vi "ManualControls_v4.vi"() -> ()   [LabVIEW 2013]
uses:
  <vilib>/Utility/miscctls.llb/LVPointTypeDef.ctl
  <vilib>/DAQmx/write.llb/DAQmx Write (Analog DBL 1Chan 1Samp).vi
  <vilib>/DAQmx/write.llb/DAQmx Write (Digital U32 1Chan 1Samp).vi
  <vilib>/DAQmx/miscellaneous.llb/DAQmx Fill In Error Info.vi
  DeviceVIs/Novatech/Novatech 409A.lvlib
panel:
  in  "Update Hardware":bool
  in  "?":enum32{"Controls", "File IO", "Errors"}(tab)
  in  "Master Output Bits":bool[](array[boolean])=[TRUE, TRUE, TRUE, TRUE, FALSE, FALSE, TRUE, FALSE, FALSE, FALSE, TRUE, FALSE, TRUE, TRUE, TRUE, TRUE, FALSE, FALSE, FALSE, FALSE, FALSE, FALSE, FALSE, FALSE]
  in  "Slave Output Bits":bool[](array[boolean])=[FALSE, FALSE, FALSE, FALSE, FALSE, FALSE, FALSE, FALSE, FALSE, FALSE, FALSE, FALSE, FALSE, FALSE, FALSE, FALSE, FALSE, FALSE, FALSE, FALSE, FALSE, FALSE, FALSE, FALSE]
  in  "Set Master":bool=TRUE
  in  "Set Slave":bool
  in  "AO Values":T1(array[cluster])=[{"DAQmx Global Channel"="AO0_0", "Numeric"=-9.792}, {"DAQmx Global Channel"="AO0_1", "Numeric"=-7.904}, {"DAQmx Global Channel"="AO0_2", "Numeric"=-3.981}, {"DAQmx Global Channel"="AO0_3", "Numeric"=-7.5}, {"DAQmx Global Channel"="AO0_4", "Numeric"=7.0}, {"DAQmx Global Channel"="AO0_5", "Numeric"=1.18}, {"DAQmx Global Channel"="AO0_6", "Numeric"=-8.918}, {"DAQmx Global Channel"="AO0_7", "Numeric"=1.1}, {"DAQmx Global Channel"="AO1_0", "Numeric"=8.0}, {"DAQmx Global Channel"="AO1_1", "Numeric"=0.45}, {"DAQmx Global Channel"="AO1_2", "Numeric"=1.3}, {"DAQmx Global Channel"="AO1_3", "Numeric"=0.0}, {"DAQmx Global Channel"="AO1_4", "Numeric"=0.3}, {"DAQmx Global Channel"="AO1_5", "Numeric"=1.2}, {"DAQmx Global Channel"="AO1_6", "Numeric"=1.6}, {"DAQmx Global Channel"="AO1_7", "Numeric"=0.12}, {"DAQmx Global Channel"="AO2_0", "Numeric"=0.0}, {"DAQmx Global Channel"="AO2_1", "Numeric"=0.0}, {"DAQmx Global Channel"="AO3_0", "Numeric"=0.0}, {"DAQmx Global Channel"="AO3_1", "Numeric"=0.0}, {"DAQmx Global Channel"="AO3_2", "Numeric"=0.0}, {"DAQmx Global Channel"="AO3_3", "Numeric"=0.0}, {"DAQmx Global Channel"="AO3_4", "Numeric"=0.0}, {"DAQmx Global Channel"="AO3_5", "Numeric"=0.0}, {"DAQmx Global Channel"="AO3_6", "Numeric"=0.0}, {"DAQmx Global Channel"="AO3_7", "Numeric"=0.0}] {"Numeric" step=1e-09 format="%_6g"}
  in  "Presets":T2(ring)
  in  "DO Values":T3(array[cluster])=[{"DAQmx Global Channel"="DO0_0", "DO Bits"=[TRUE, TRUE, FALSE, FALSE, FALSE, FALSE, TRUE, TRUE, FALSE, FALSE, FALSE, FALSE, FALSE, FALSE, FALSE, FALSE]}, {"DAQmx Global Channel"="DO1_0", "DO Bits"=[TRUE, FALSE, TRUE, TRUE, FALSE, TRUE, TRUE, TRUE, FALSE, FALSE, FALSE, FALSE, FALSE, FALSE, FALSE, FALSE]}, {"DAQmx Global Channel"="DO2_0", "DO Bits"=[]}, {"DAQmx Global Channel"="DO3_0", "DO Bits"=[]}]
  in  "Novatech settings":T4(array[cluster])
  in  "History":string(combo)
  in  "Save":bool
  in  "Load":bool
  in  "Path":path=path "C:/Experiment/Data Acquisition/Hardware Control/procedures/ManualControl"
  in  "error in":errorcluster
  out "error out":errorcluster
  # "Analog out"
  # "Digital Out"
  # "Ports are setup for 16 bit output, but only 16 are used"
  # "Master PB (PB 0)"
  # "Slave PB (PB 1)"
  # "Novatechs"
  # "0"
  # "8"
  # "12"
  # "4"
  # "16"
  # "20"
  # "0"
  # "8"
  # "12"
  # "4"
  # "16"
  # "20"
  # "Templates"
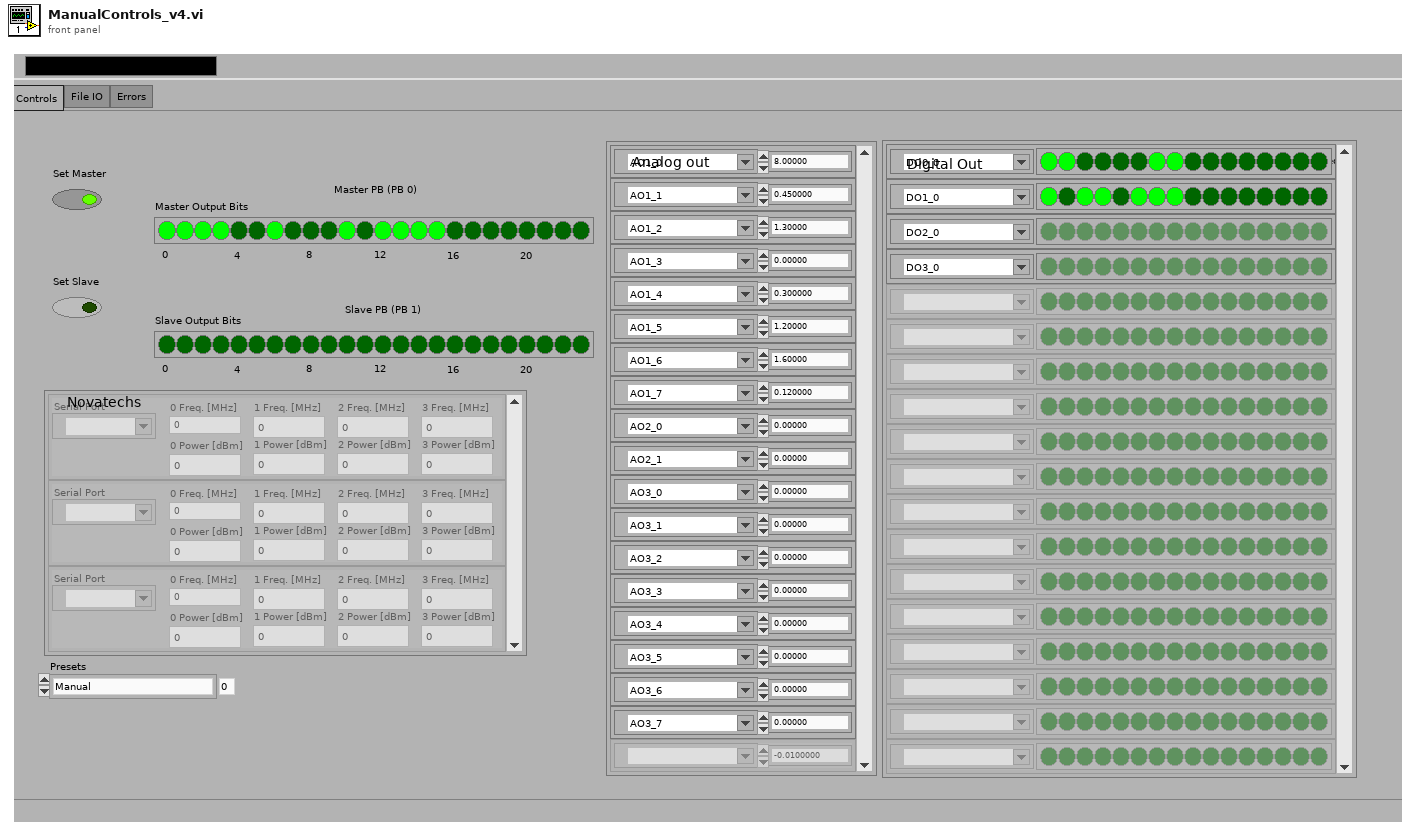
[diagram p1: front panel]
types:
  T1 = cluster{"DAQmx Global Channel":refnum<k21>, "Numeric":dbl}[]
  T2 = enum16{"Manual", "Rb MOT", "Yb MOT", "RbYb Warmup", "RbYb Turn Off", "Sr Warmup"}
  T3 = cluster{"DAQmx Global Channel":refnum<k21>, "DO Bits":bool[]}[]
  T4 = cluster{"0 Freq. [MHz]":dbl, "0 Power [dBm]":dbl, "Serial Port":refnum<visa-resource-name>, "1 Freq. [MHz]":dbl, "1 Power [dBm]":dbl, "2 Freq. [MHz]":dbl, "2 Power [dBm]":dbl, "3 Freq. [MHz]":dbl, "3 Power [dBm]":dbl}[]
  T5 = typedef "Semaphore RefNum" = refnum<k1>
  T6 = enum16{"open", "open or create", "create or replace", "create", "open (read only)"}
  T7 = enum16{"Always On", "Always Off", "Off While Running"}
  T8 = typedef "LVPointTypeDef.ctl" = cluster{"Horizontal":i16, "Vertical":i16}
  T9 = cluster{"Master Output Bits":bool[], "Slave Output Bits":bool[], "AO Values":cluster{"DAQmx Global Channel":refnum<k21>, "Numeric":dbl}[], "DO Values":cluster{"DAQmx Global Channel":refnum<k21>, "DO Bits":bool[]}[], "Novatech settings":cluster{"0 Freq. [MHz]":dbl, "0 Power [dBm]":dbl, "Serial Port":refnum<visa-resource-name>, "1 Freq. [MHz]":dbl, "1 Power [dBm]":dbl, "2 Freq. [MHz]":dbl, "2 Power [dBm]":dbl, "3 Freq. [MHz]":dbl, "3 Power [dBm]":dbl}[]}
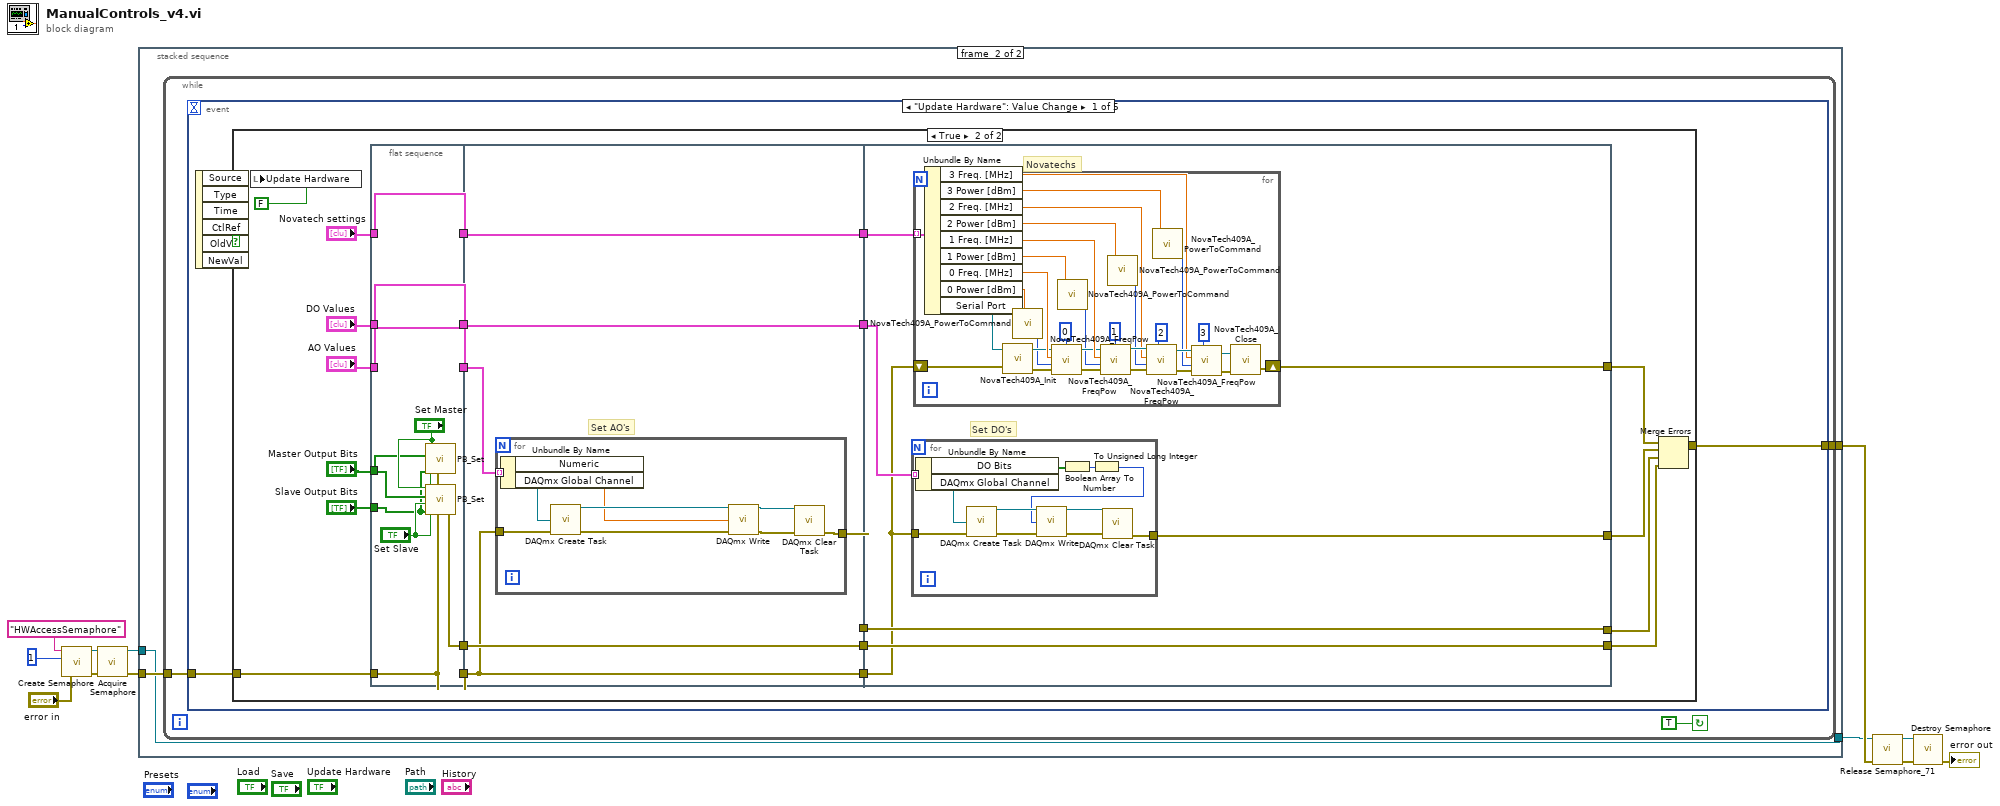
[diagram p0: block diagram]
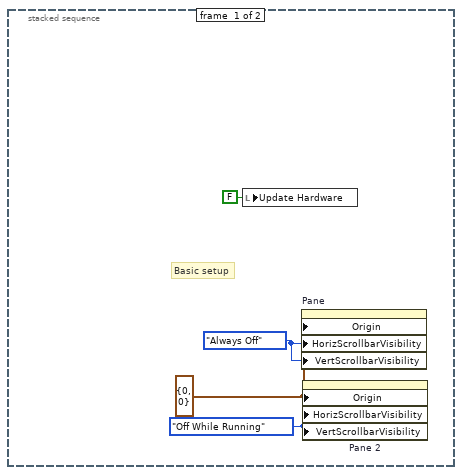
[diagram p2: hidden frame]
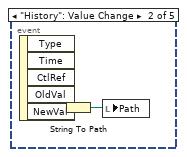
[diagram p4: hidden frame]
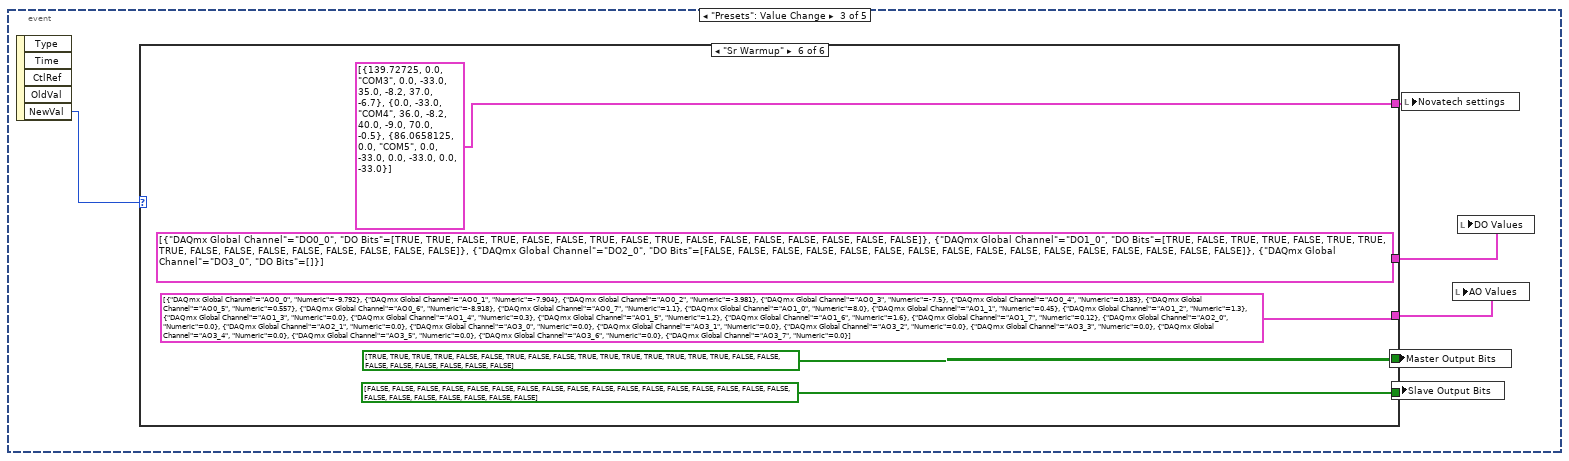
[diagram p5: hidden frame]
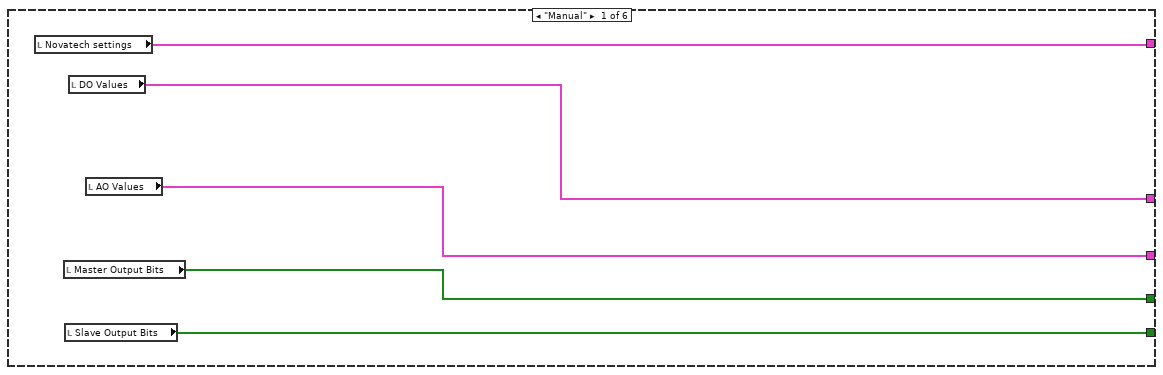
[diagram p6: hidden frame]
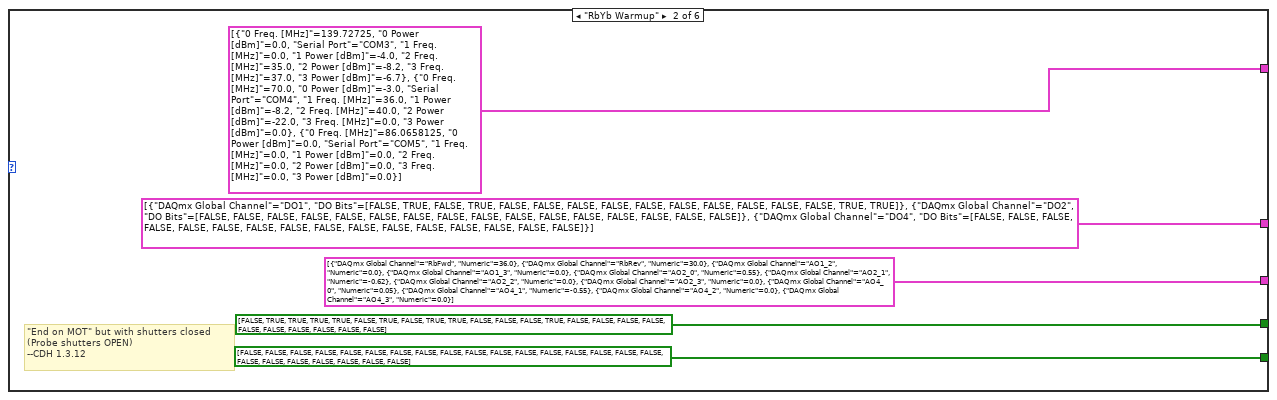
[diagram p7: hidden frame]
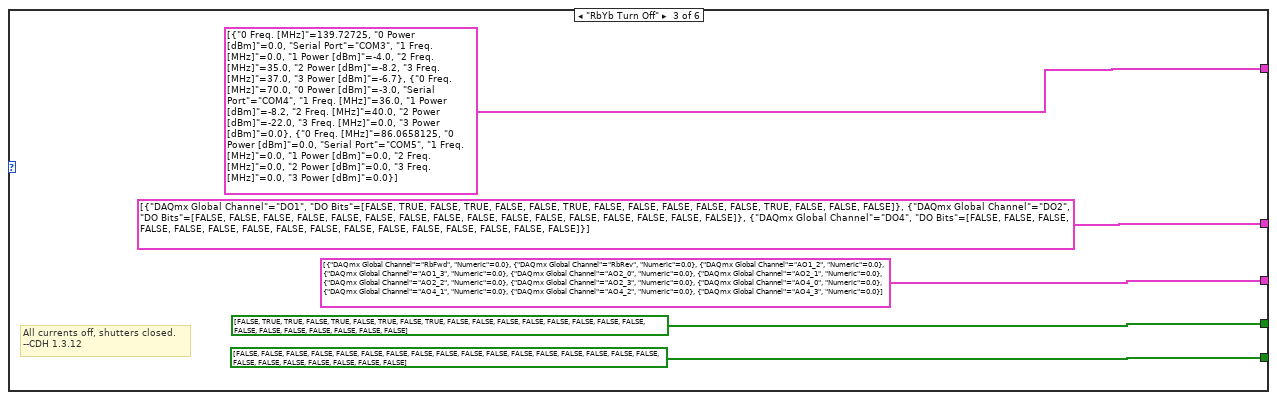
[diagram p8: hidden frame]
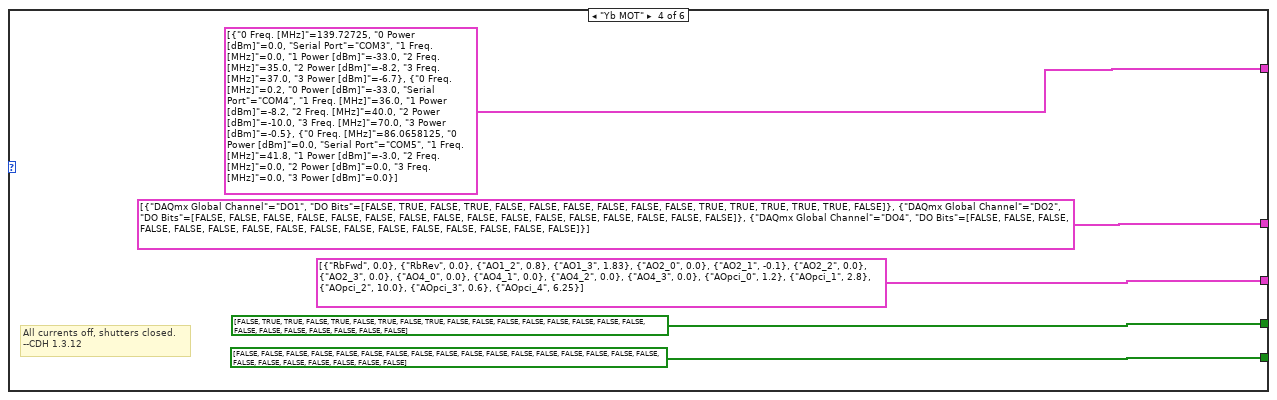
[diagram p9: hidden frame]
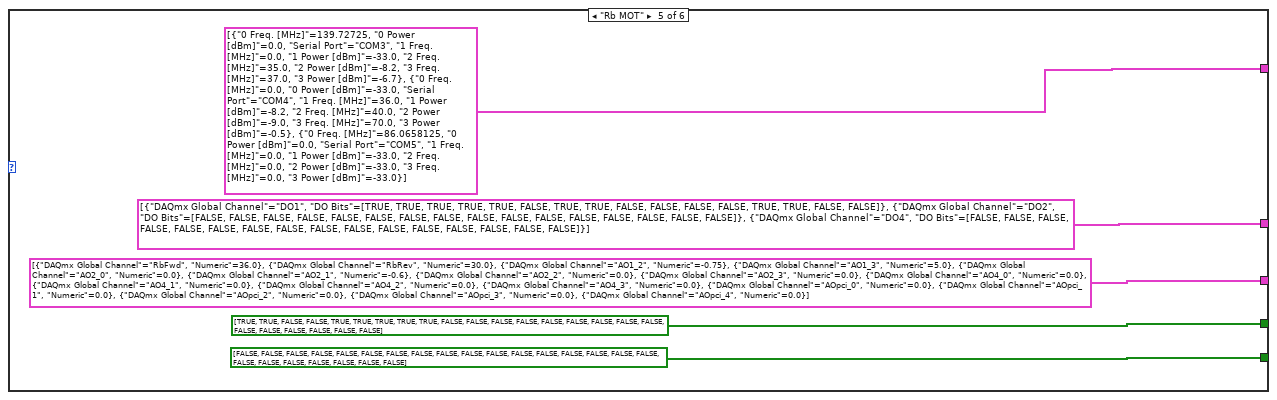
[diagram p10: hidden frame]
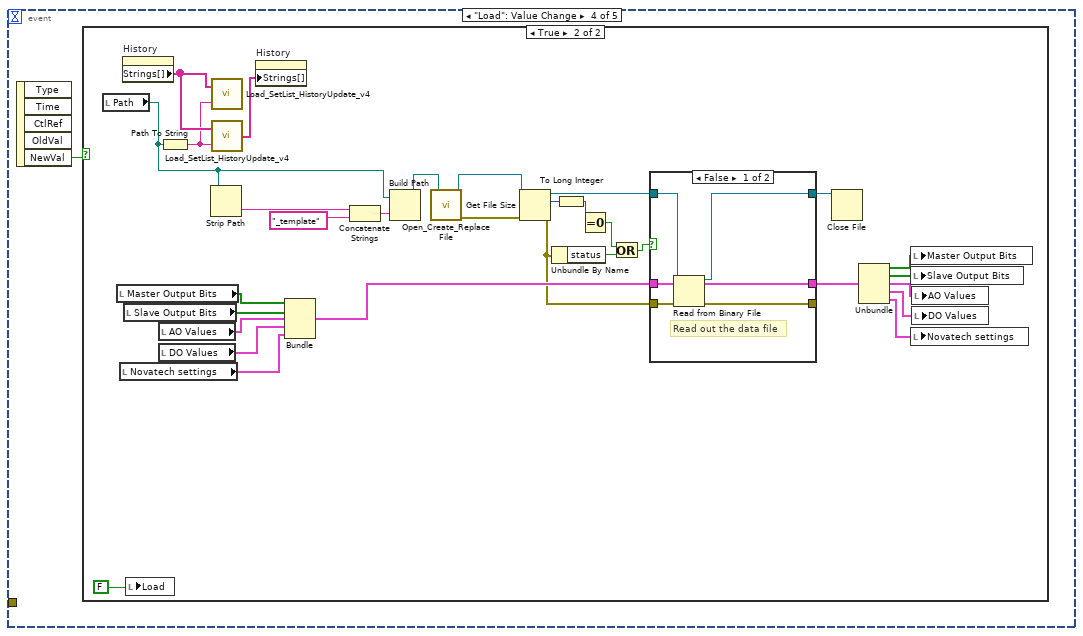
[diagram p11: hidden frame]
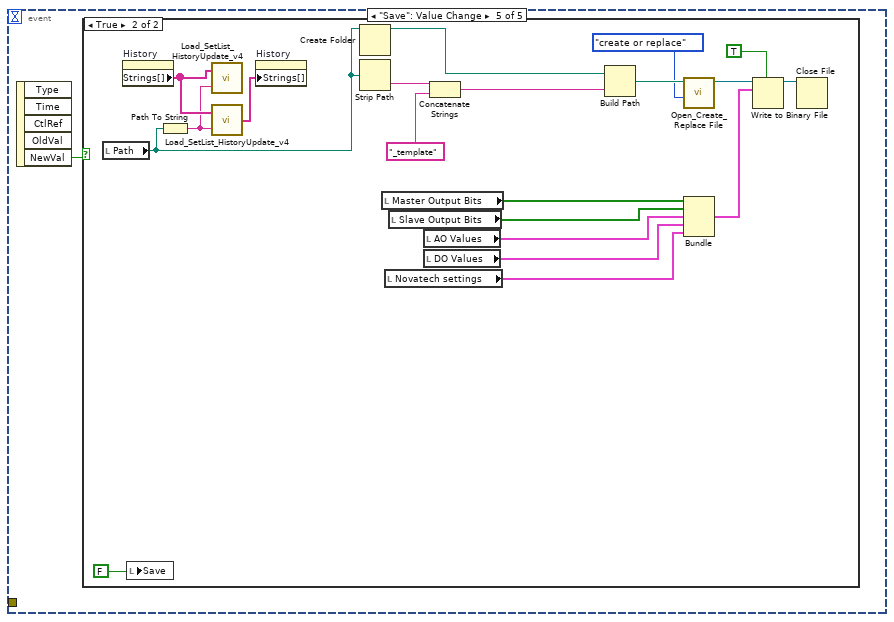
[diagram p14: hidden frame]
diagram:
  n1 = call <vilib>:"Create Semaphore.vi"("error in (no error)"="error in", "size (1)"=1, "name (unnamed)"="HWAccessSemaphore") -> ("error out"=w6:errorcluster, "semaphore"=w7:T5)  [unwired: 3 out]
  n2 = call <vilib>:"Acquire Semaphore.vi"("error in (no error)"=w6, "semaphore"=w7) -> ("error out"=w3:errorcluster, "semaphore out"=w2:T5)  [unwired: 1 in, 3 out]
  n3 = stacked-sequence {
    tunnel: [_ w19] -> w9
    tunnel: w3 -> [_ w18]
    tunnel: w2 -> [_ w17]
    tunnel: [_ w17] -> w1
    frame #0 {
      w16 = T7."Always Off" ("Horizontal Scrollbar Visibility")
      w15 = T8 {"Horizontal"=0, "Vertical"=0} ("Origin")
      w14 = T7."Off While Running" ("Horizontal Scrollbar Visibility")
      # "Basic setup"
      n4 = local write "Update Hardware"(FALSE ("Update Hardware")) -> ()
      n5 = property on="Pane" class="Pane"("Origin"=w15, "HorizScrollbarVisibility"=w16, "VertScrollbarVisibility"=w16) -> ()  [unwired: 2 in, 2 out]
      n6 = property on="Pane 2" class="Pane"("Origin"=w15, "HorizScrollbarVisibility"=w14, "VertScrollbarVisibility"=w14) -> ()  [unwired: 2 in, 2 out]
    }
    frame #1 {
      n7 = while {
        tunnel: [w22] -> w19
        tunnel: w18 -> [w21]
        stop <- TRUE continue-if-true
        n8 = event shown="[0] \"Update Hardware\": Value Change" {
          selector: _ -> [_ _ _ _ _]
          dyn-events: _ -> [_ _ _ _ _]
          timeout: _ -> [_ _ _ _ _]
          tunnel: [w25 _ _ _ _] -> w22
          tunnel: w21 -> [w24 _ _ _ _]
          event "Update Hardware": Value Change {
            n9 = event-data() -> ("OldVal"=w23:bool)  [unwired: 1 in, 5 out]
            n10 = case shown="True" w23 {
              tunnel: [w26 w36] -> w25
              tunnel: w24 -> [w26 w35]
              frame False {
              }
              frame True {
                n11 = local write "Update Hardware"(FALSE) -> ()
                n12 = flat-sequence {
                  tunnel: [w49] -> w48
                  tunnel: [w55] -> w47
                  tunnel: "AO Values" -> [w55]
                  tunnel: "Master Output Bits" -> [w54]
                  tunnel: "Slave Output Bits" -> [w53]
                  tunnel: "DO Values" -> [w51]
                  tunnel: "Novatech settings" -> [w52]
                  tunnel: [w51] -> w46
                  tunnel: [w52] -> w45
                  tunnel: w35 -> [w50]
                  tunnel: [w50] -> w44
                  tunnel: w48 -> [w59]
                  tunnel: w47 -> [w62]
                  tunnel: [w63] -> w43
                  tunnel: w46 -> [w61]
                  tunnel: [w61] -> w42
                  tunnel: [w60] -> w41
                  tunnel: w45 -> [w60]
                  tunnel: [w58] -> w40
                  tunnel: w44 -> [w58]
                  tunnel: [w59] -> w39
                  tunnel: [w79] -> w37
                  tunnel: w43 -> [w74]
                  tunnel: w42 -> [w78]
                  tunnel: [w77] -> w38
                  tunnel: w41 -> [w76]
                  tunnel: w40 -> [w73]
                  tunnel: [w75] -> w28
                  tunnel: w39 -> [w75]
                  tunnel: [w74] -> w29
                  frame #0 {
                    # "Set PulseBlaster"
                    n13 = call "PB_Set.vi"("Set Master"="Set Master", "Master Output Bits"=w54, "Set Slave"="Set Slave", "Slave Output Bits"=w53, "error in"=w50) -> ()  [unwired: 3 out]
                    n14 = call "PB_Set.vi"("Set Master"="Set Master", "Master Output Bits"=w54, "Set Slave"="Set Slave", "Slave Output Bits"=w53, "error in"=w50) -> ("error out"=w49:errorcluster)  [unwired: 2 out]
                  }
                  frame #1 {
                    # "Set AO's"
                    n15 = for {
                      tunnel: [w70] -> w63
                      tunnel: w58 -> [w69]
                      tunnel: w62 -> [w66] mode=indexing
                      n16 = Unbundle By Name(w66) -> ("Numeric"=w65:dbl, "DAQmx Global Channel"=w64:refnum<k21>)
                      n17 = call <vilib>:"DAQmx Create Task.vi"("global virtual channels"=w64, "error in"=w69) -> ("task out"=w67:refnum<k21>, "error out"=w68:errorcluster)  [unwired: 3 in, 9 out]
                      n18 = call-poly <vilib>:"DAQmx Write.vi"("task/channels in"=w67, "data"=w65, "error in"=w68) -> ("task out"=w72:refnum<k21>, "error out"=w71:errorcluster)  [unwired: 1 in, 10 out]
                      n19 = call <vilib>:"DAQmx Clear Task.vi"("task in"=w72, "error in"=w71) -> ("error out"=w70:errorcluster)  [unwired: 13 out]
                    }
                  }
                  frame #2 {
                    # "Novatechs"
                    # "Set DO's"
                    n20 = for {
                      tunnel: [w118] -> w79
                      tunnel: w73 -> [w117]
                      tunnel: w78 -> [w114] mode=indexing
                      n21 = Unbundle By Name(w114) -> ("DO Bits"=w111:bool[], "DAQmx Global Channel"=w113:refnum<k21>)
                      n22 = call <vilib>:"DAQmx Create Task.vi"("global virtual channels"=w113, "error in"=w117) -> ("task out"=w115:refnum<k21>, "error out"=w116:errorcluster)  [unwired: 3 in, 9 out]
                      n23 = Boolean Array To Number(Boolean array=w111) -> (number=w112:u32)
                      n24 = To Unsigned Long Integer(number=w112) -> (unsigned 32bit integer=w110:u32)
                      n25 = call-poly <vilib>:"DAQmx Write.vi"("task/channels in"=w115, "data"=w110, "error in"=w116) -> ("task out"=w120:refnum<k21>, "error out"=w119:errorcluster)  [unwired: 1 in, 10 out]
                      n26 = call <vilib>:"DAQmx Clear Task.vi"("task in"=w120, "error in"=w119) -> ("error out"=w118:errorcluster)  [unwired: 13 out]
                    }
                    n27 = for {
                      tunnel: w76 -> [w109] mode=indexing
                      shift-right: [w95] -> w77
                      shift-left: w73 -> [w107]
                      n28 = Unbundle By Name(w109) -> ("3 Freq. [MHz]"=w88:dbl, "3 Power [dBm]"=w87:dbl, "2 Freq. [MHz]"=w89:dbl, "2 Power [dBm]"=w84:dbl, "1 Freq. [MHz]"=w102:dbl, "1 Power [dBm]"=w82:dbl, "0 Freq. [MHz]"=w104:dbl, "0 Power [dBm]"=w80:dbl, "Serial Port"=w108:refnum<visa-resource-name>)
                      n29 = call "NovaTech409A_Init.vi"("error in (no error)"=w107, "VISA resource name"=w108) -> ("error out"=w106:errorcluster, "VISA resource name out"=w103:refnum<visa-resource-name>)  [unwired: 1 in]
                      n30 = call "NovaTech409A_PowerToCommand.vi"("Novatech Power [dBm]"=w80) -> ("Novatech Command"=w81:u16)
                      n31 = call "NovaTech409A_FreqPow.vi"("VISA resource name"=w103, "Freq"=w104, "Power"=w81, "error in (no error)"=w106, "Channel (0-3)"=u8 0) -> ("VISA resource name out"=w101:refnum<visa-resource-name>, "error out"=w105:errorcluster)
                      n32 = call "NovaTech409A_PowerToCommand.vi"("Novatech Power [dBm]"=w82) -> ("Novatech Command"=w83:u16)
                      n33 = call "NovaTech409A_FreqPow.vi"("VISA resource name"=w101, "Freq"=w102, "Power"=w83, "error in (no error)"=w105, "Channel (0-3)"=u8 1) -> ("VISA resource name out"=w94:refnum<visa-resource-name>, "error out"=w98:errorcluster)
                      n34 = call "NovaTech409A_PowerToCommand.vi"("Novatech Power [dBm]"=w84) -> ("Novatech Command"=w85:u16)
                      n35 = call "NovaTech409A_FreqPow.vi"("VISA resource name"=w94, "Freq"=w89, "Power"=w85, "error in (no error)"=w98, "Channel (0-3)"=u8 2) -> ("VISA resource name out"=w93:refnum<visa-resource-name>, "error out"=w97:errorcluster)
                      n36 = call "NovaTech409A_PowerToCommand.vi"("Novatech Power [dBm]"=w87) -> ("Novatech Command"=w86:u16)
                      n37 = call "NovaTech409A_FreqPow.vi"("VISA resource name"=w93, "Freq"=w88, "Power"=w86, "error in (no error)"=w97, "Channel (0-3)"=u8 3) -> ("VISA resource name out"=w92:refnum<visa-resource-name>, "error out"=w96:errorcluster)
                      n38 = call "NovaTech409A_Close.vi"("error in (no error)"=w96, "VISA resource name"=w92) -> ("error out"=w95:errorcluster)  [unwired: 1 out]
                    }
                  }
                }
                n39 = Merge Errors(w38, w37, w29, w28) -> (w36:errorcluster)
              }
            }
          }
          event "History": Value Change {
            n40 = event-data() -> ("NewVal"=w122:string)  [unwired: 1 in, 4 out]
            n41 = String To Path(string=w122) -> (path=w121:path)
            n42 = local write "Path"(w121) -> ()
          }
          event "Presets": Value Change {
            n43 = event-data() -> ("NewVal"=w123:T2)  [unwired: 1 in, 4 out]
            n44 = case shown="\"Sr Warmup\"" w123 {
              tunnel: [w131 T1 [{"DAQmx Global Channel"="RbFwd", "Numeric"=36.0}, {"DAQmx Global Channel"="RbRev", "Numeric"=30.0}, {"DAQmx Global Channel"="AO1_2", "Numeric"=0.0}, {"DAQmx Global Channel"="AO1_3", "Numeric"=0.0}, {"DAQmx Global Channel"="AO2_0", "Numeric"=0.55}, {"DAQmx Global Channel"="AO2_1", "Numeric"=-0.62}, {"DAQmx Global Channel"="AO2_2", "Numeric"=0.0}, {"DAQmx Global Channel"="AO2_3", "Numeric"=0.0}, {"DAQmx Global Channel"="AO4_0", "Numeric"=0.05}, {"DAQmx Global Channel"="AO4_1", "Numeric"=-0.55}, {"DAQmx Global Channel"="AO4_2", "Numeric"=0.0}, {"DAQmx Global Channel"="AO4_3", "Numeric"=0.0}] ("AO Values") T1 [{"DAQmx Global Channel"="RbFwd", "Numeric"=0.0}, {"DAQmx Global Channel"="RbRev", "Numeric"=0.0}, {"DAQmx Global Channel"="AO1_2", "Numeric"=0.0}, {"DAQmx Global Channel"="AO1_3", "Numeric"=0.0}, {"DAQmx Global Channel"="AO2_0", "Numeric"=0.0}, {"DAQmx Global Channel"="AO2_1", "Numeric"=0.0}, {"DAQmx Global Channel"="AO2_2", "Numeric"=0.0}, {"DAQmx Global Channel"="AO2_3", "Numeric"=0.0}, {"DAQmx Global Channel"="AO4_0", "Numeric"=0.0}, {"DAQmx Global Channel"="AO4_1", "Numeric"=0.0}, {"DAQmx Global Channel"="AO4_2", "Numeric"=0.0}, {"DAQmx Global Channel"="AO4_3", "Numeric"=0.0}] ("AO Values") T1 [{"DAQmx Global Channel"="RbFwd", "Numeric"=0.0}, {"DAQmx Global Channel"="RbRev", "Numeric"=0.0}, {"DAQmx Global Channel"="AO1_2", "Numeric"=0.8}, {"DAQmx Global Channel"="AO1_3", "Numeric"=1.83}, {"DAQmx Global Channel"="AO2_0", "Numeric"=0.0}, {"DAQmx Global Channel"="AO2_1", "Numeric"=-0.1}, {"DAQmx Global Channel"="AO2_2", "Numeric"=0.0}, {"DAQmx Global Channel"="AO2_3", "Numeric"=0.0}, {"DAQmx Global Channel"="AO4_0", "Numeric"=0.0}, {"DAQmx Global Channel"="AO4_1", "Numeric"=0.0}, {"DAQmx Global Channel"="AO4_2", "Numeric"=0.0}, {"DAQmx Global Channel"="AO4_3", "Numeric"=0.0}, {"DAQmx Global Channel"="AOpci_0", "Numeric"=1.2}, {"DAQmx Global Channel"="AOpci_1", "Numeric"=2.8}, {"DAQmx Global Channel"="AOpci_2", "Numeric"=10.0}, {"DAQmx Global Channel"="AOpci_3", "Numeric"=0.6}, {"DAQmx Global Channel"="AOpci_4", "Numeric"=6.25}] ("AO Values") T1 [{"DAQmx Global Channel"="RbFwd", "Numeric"=36.0}, {"DAQmx Global Channel"="RbRev", "Numeric"=30.0}, {"DAQmx Global Channel"="AO1_2", "Numeric"=-0.75}, {"DAQmx Global Channel"="AO1_3", "Numeric"=5.0}, {"DAQmx Global Channel"="AO2_0", "Numeric"=0.0}, {"DAQmx Global Channel"="AO2_1", "Numeric"=-0.6}, {"DAQmx Global Channel"="AO2_2", "Numeric"=0.0}, {"DAQmx Global Channel"="AO2_3", "Numeric"=0.0}, {"DAQmx Global Channel"="AO4_0", "Numeric"=0.0}, {"DAQmx Global Channel"="AO4_1", "Numeric"=0.0}, {"DAQmx Global Channel"="AO4_2", "Numeric"=0.0}, {"DAQmx Global Channel"="AO4_3", "Numeric"=0.0}, {"DAQmx Global Channel"="AOpci_0", "Numeric"=0.0}, {"DAQmx Global Channel"="AOpci_1", "Numeric"=0.0}, {"DAQmx Global Channel"="AOpci_2", "Numeric"=0.0}, {"DAQmx Global Channel"="AOpci_3", "Numeric"=0.0}, {"DAQmx Global Channel"="AOpci_4", "Numeric"=0.0}] ("AO Values") T1 [{"DAQmx Global Channel"="AO0_0", "Numeric"=-9.792}, {"DAQmx Global Channel"="AO0_1", "Numeric"=-7.904}, {"DAQmx Global Channel"="AO0_2", "Numeric"=-3.981}, {"DAQmx Global Channel"="AO0_3", "Numeric"=-7.5}, {"DAQmx Global Channel"="AO0_4", "Numeric"=0.183}, {"DAQmx Global Channel"="AO0_5", "Numeric"=0.557}, {"DAQmx Global Channel"="AO0_6", "Numeric"=-8.918}, {"DAQmx Global Channel"="AO0_7", "Numeric"=1.1}, {"DAQmx Global Channel"="AO1_0", "Numeric"=8.0}, {"DAQmx Global Channel"="AO1_1", "Numeric"=0.45}, {"DAQmx Global Channel"="AO1_2", "Numeric"=1.3}, {"DAQmx Global Channel"="AO1_3", "Numeric"=0.0}, {"DAQmx Global Channel"="AO1_4", "Numeric"=0.3}, {"DAQmx Global Channel"="AO1_5", "Numeric"=1.2}, {"DAQmx Global Channel"="AO1_6", "Numeric"=1.6}, {"DAQmx Global Channel"="AO1_7", "Numeric"=0.12}, {"DAQmx Global Channel"="AO2_0", "Numeric"=0.0}, {"DAQmx Global Channel"="AO2_1", "Numeric"=0.0}, {"DAQmx Global Channel"="AO3_0", "Numeric"=0.0}, {"DAQmx Global Channel"="AO3_1", "Numeric"=0.0}, {"DAQmx Global Channel"="AO3_2", "Numeric"=0.0}, {"DAQmx Global Channel"="AO3_3", "Numeric"=0.0}, {"DAQmx Global Channel"="AO3_4", "Numeric"=0.0}, {"DAQmx Global Channel"="AO3_5", "Numeric"=0.0}, {"DAQmx Global Channel"="AO3_6", "Numeric"=0.0}, {"DAQmx Global Channel"="AO3_7", "Numeric"=0.0}] ("AO Values")] -> w126
              tunnel: [w130 bool[] [FALSE, TRUE, TRUE, TRUE, TRUE, FALSE, TRUE, FALSE, TRUE, TRUE, FALSE, FALSE, FALSE, TRUE, FALSE, FALSE, FALSE, FALSE, FALSE, FALSE, FALSE, FALSE, FALSE, FALSE] ("Master Output Bits") bool[] [FALSE, TRUE, TRUE, FALSE, TRUE, FALSE, TRUE, FALSE, TRUE, FALSE, FALSE, FALSE, FALSE, FALSE, FALSE, FALSE, FALSE, FALSE, FALSE, FALSE, FALSE, FALSE, FALSE, FALSE] ("Master Output Bits") bool[] [FALSE, TRUE, TRUE, FALSE, TRUE, FALSE, TRUE, FALSE, TRUE, FALSE, FALSE, FALSE, FALSE, FALSE, FALSE, FALSE, FALSE, FALSE, FALSE, FALSE, FALSE, FALSE, FALSE, FALSE] ("Master Output Bits") bool[] [TRUE, TRUE, FALSE, FALSE, TRUE, TRUE, TRUE, TRUE, TRUE, FALSE, FALSE, FALSE, FALSE, FALSE, FALSE, FALSE, FALSE, FALSE, FALSE, FALSE, FALSE, FALSE, FALSE, FALSE] ("Master Output Bits") bool[] [TRUE, TRUE, TRUE, TRUE, FALSE, FALSE, TRUE, FALSE, FALSE, TRUE, TRUE, TRUE, TRUE, TRUE, TRUE, TRUE, FALSE, FALSE, FALSE, FALSE, FALSE, FALSE, FALSE, FALSE] ("Master Output Bits")] -> w124
              tunnel: [w129 bool[] [FALSE, FALSE, FALSE, FALSE, FALSE, FALSE, FALSE, FALSE, FALSE, FALSE, FALSE, FALSE, FALSE, FALSE, FALSE, FALSE, FALSE, FALSE, FALSE, FALSE, FALSE, FALSE, FALSE, FALSE] ("Slave Output Bits") bool[] [FALSE, FALSE, FALSE, FALSE, FALSE, FALSE, FALSE, FALSE, FALSE, FALSE, FALSE, FALSE, FALSE, FALSE, FALSE, FALSE, FALSE, FALSE, FALSE, FALSE, FALSE, FALSE, FALSE, FALSE] ("Slave Output Bits") bool[] [FALSE, FALSE, FALSE, FALSE, FALSE, FALSE, FALSE, FALSE, FALSE, FALSE, FALSE, FALSE, FALSE, FALSE, FALSE, FALSE, FALSE, FALSE, FALSE, FALSE, FALSE, FALSE, FALSE, FALSE] ("Slave Output Bits") bool[] [FALSE, FALSE, FALSE, FALSE, FALSE, FALSE, FALSE, FALSE, FALSE, FALSE, FALSE, FALSE, FALSE, FALSE, FALSE, FALSE, FALSE, FALSE, FALSE, FALSE, FALSE, FALSE, FALSE, FALSE] ("Slave Output Bits") bool[] [FALSE, FALSE, FALSE, FALSE, FALSE, FALSE, FALSE, FALSE, FALSE, FALSE, FALSE, FALSE, FALSE, FALSE, FALSE, FALSE, FALSE, FALSE, FALSE, FALSE, FALSE, FALSE, FALSE, FALSE] ("Slave Output Bits")] -> w125
              tunnel: [w132 T3 [{"DAQmx Global Channel"="DO1", "DO Bits"=[FALSE, TRUE, FALSE, TRUE, FALSE, FALSE, FALSE, FALSE, FALSE, FALSE, FALSE, FALSE, FALSE, FALSE, TRUE, TRUE]}, {"DAQmx Global Channel"="DO2", "DO Bits"=[FALSE, FALSE, FALSE, FALSE, FALSE, FALSE, FALSE, FALSE, FALSE, FALSE, FALSE, FALSE, FALSE, FALSE, FALSE, FALSE]}, {"DAQmx Global Channel"="DO4", "DO Bits"=[FALSE, FALSE, FALSE, FALSE, FALSE, FALSE, FALSE, FALSE, FALSE, FALSE, FALSE, FALSE, FALSE, FALSE, FALSE, FALSE]}] ("DO Values") T3 [{"DAQmx Global Channel"="DO1", "DO Bits"=[FALSE, TRUE, FALSE, TRUE, FALSE, FALSE, TRUE, FALSE, FALSE, FALSE, FALSE, FALSE, TRUE, FALSE, FALSE, FALSE]}, {"DAQmx Global Channel"="DO2", "DO Bits"=[FALSE, FALSE, FALSE, FALSE, FALSE, FALSE, FALSE, FALSE, FALSE, FALSE, FALSE, FALSE, FALSE, FALSE, FALSE, FALSE]}, {"DAQmx Global Channel"="DO4", "DO Bits"=[FALSE, FALSE, FALSE, FALSE, FALSE, FALSE, FALSE, FALSE, FALSE, FALSE, FALSE, FALSE, FALSE, FALSE, FALSE, FALSE]}] ("DO Values") T3 [{"DAQmx Global Channel"="DO1", "DO Bits"=[FALSE, TRUE, FALSE, TRUE, FALSE, FALSE, FALSE, FALSE, FALSE, FALSE, TRUE, TRUE, TRUE, TRUE, TRUE, FALSE]}, {"DAQmx Global Channel"="DO2", "DO Bits"=[FALSE, FALSE, FALSE, FALSE, FALSE, FALSE, FALSE, FALSE, FALSE, FALSE, FALSE, FALSE, FALSE, FALSE, FALSE, FALSE]}, {"DAQmx Global Channel"="DO4", "DO Bits"=[FALSE, FALSE, FALSE, FALSE, FALSE, FALSE, FALSE, FALSE, FALSE, FALSE, FALSE, FALSE, FALSE, FALSE, FALSE, FALSE]}] ("DO Values") T3 [{"DAQmx Global Channel"="DO1", "DO Bits"=[TRUE, TRUE, TRUE, TRUE, TRUE, FALSE, TRUE, TRUE, FALSE, FALSE, FALSE, FALSE, TRUE, TRUE, FALSE, FALSE]}, {"DAQmx Global Channel"="DO2", "DO Bits"=[FALSE, FALSE, FALSE, FALSE, FALSE, FALSE, FALSE, FALSE, FALSE, FALSE, FALSE, FALSE, FALSE, FALSE, FALSE, FALSE]}, {"DAQmx Global Channel"="DO4", "DO Bits"=[FALSE, FALSE, FALSE, FALSE, FALSE, FALSE, FALSE, FALSE, FALSE, FALSE, FALSE, FALSE, FALSE, FALSE, FALSE, FALSE]}] ("DO Values") T3 [{"DAQmx Global Channel"="DO0_0", "DO Bits"=[TRUE, TRUE, FALSE, TRUE, FALSE, FALSE, TRUE, FALSE, TRUE, FALSE, FALSE, FALSE, FALSE, FALSE, FALSE, FALSE]}, {"DAQmx Global Channel"="DO1_0", "DO Bits"=[TRUE, FALSE, TRUE, TRUE, FALSE, TRUE, TRUE, TRUE, FALSE, FALSE, FALSE, FALSE, FALSE, FALSE, FALSE, FALSE]}, {"DAQmx Global Channel"="DO2_0", "DO Bits"=[FALSE, FALSE, FALSE, FALSE, FALSE, FALSE, FALSE, FALSE, FALSE, FALSE, FALSE, FALSE, FALSE, FALSE, FALSE, FALSE]}, {"DAQmx Global Channel"="DO3_0", "DO Bits"=[]}] ("DO Values")] -> w127
              tunnel: [w133 T4 [{"0 Freq. [MHz]"=139.72725, "0 Power [dBm]"=0.0, "Serial Port"="COM3", "1 Freq. [MHz]"=0.0, "1 Power [dBm]"=-4.0, "2 Freq. [MHz]"=35.0, "2 Power [dBm]"=-8.2, "3 Freq. [MHz]"=37.0, "3 Power [dBm]"=-6.7}, {"0 Freq. [MHz]"=70.0, "0 Power [dBm]"=-3.0, "Serial Port"="COM4", "1 Freq. [MHz]"=36.0, "1 Power [dBm]"=-8.2, "2 Freq. [MHz]"=40.0, "2 Power [dBm]"=-22.0, "3 Freq. [MHz]"=0.0, "3 Power [dBm]"=0.0}, {"0 Freq. [MHz]"=86.0658125, "0 Power [dBm]"=0.0, "Serial Port"="COM5", "1 Freq. [MHz]"=0.0, "1 Power [dBm]"=0.0, "2 Freq. [MHz]"=0.0, "2 Power [dBm]"=0.0, "3 Freq. [MHz]"=0.0, "3 Power [dBm]"=0.0}] ("Novatech settings") T4 [{"0 Freq. [MHz]"=139.72725, "0 Power [dBm]"=0.0, "Serial Port"="COM3", "1 Freq. [MHz]"=0.0, "1 Power [dBm]"=-4.0, "2 Freq. [MHz]"=35.0, "2 Power [dBm]"=-8.2, "3 Freq. [MHz]"=37.0, "3 Power [dBm]"=-6.7}, {"0 Freq. [MHz]"=70.0, "0 Power [dBm]"=-3.0, "Serial Port"="COM4", "1 Freq. [MHz]"=36.0, "1 Power [dBm]"=-8.2, "2 Freq. [MHz]"=40.0, "2 Power [dBm]"=-22.0, "3 Freq. [MHz]"=0.0, "3 Power [dBm]"=0.0}, {"0 Freq. [MHz]"=86.0658125, "0 Power [dBm]"=0.0, "Serial Port"="COM5", "1 Freq. [MHz]"=0.0, "1 Power [dBm]"=0.0, "2 Freq. [MHz]"=0.0, "2 Power [dBm]"=0.0, "3 Freq. [MHz]"=0.0, "3 Power [dBm]"=0.0}] ("Novatech settings") T4 [{"0 Freq. [MHz]"=139.72725, "0 Power [dBm]"=0.0, "Serial Port"="COM3", "1 Freq. [MHz]"=0.0, "1 Power [dBm]"=-33.0, "2 Freq. [MHz]"=35.0, "2 Power [dBm]"=-8.2, "3 Freq. [MHz]"=37.0, "3 Power [dBm]"=-6.7}, {"0 Freq. [MHz]"=0.2, "0 Power [dBm]"=-33.0, "Serial Port"="COM4", "1 Freq. [MHz]"=36.0, "1 Power [dBm]"=-8.2, "2 Freq. [MHz]"=40.0, "2 Power [dBm]"=-10.0, "3 Freq. [MHz]"=70.0, "3 Power [dBm]"=-0.5}, {"0 Freq. [MHz]"=86.0658125, "0 Power [dBm]"=0.0, "Serial Port"="COM5", "1 Freq. [MHz]"=41.8, "1 Power [dBm]"=-3.0, "2 Freq. [MHz]"=0.0, "2 Power [dBm]"=0.0, "3 Freq. [MHz]"=0.0, "3 Power [dBm]"=0.0}] ("Novatech settings") T4 [{"0 Freq. [MHz]"=139.72725, "0 Power [dBm]"=0.0, "Serial Port"="COM3", "1 Freq. [MHz]"=0.0, "1 Power [dBm]"=-33.0, "2 Freq. [MHz]"=35.0, "2 Power [dBm]"=-8.2, "3 Freq. [MHz]"=37.0, "3 Power [dBm]"=-6.7}, {"0 Freq. [MHz]"=0.0, "0 Power [dBm]"=-33.0, "Serial Port"="COM4", "1 Freq. [MHz]"=36.0, "1 Power [dBm]"=-8.2, "2 Freq. [MHz]"=40.0, "2 Power [dBm]"=-9.0, "3 Freq. [MHz]"=70.0, "3 Power [dBm]"=-0.5}, {"0 Freq. [MHz]"=86.0658125, "0 Power [dBm]"=0.0, "Serial Port"="COM5", "1 Freq. [MHz]"=0.0, "1 Power [dBm]"=-33.0, "2 Freq. [MHz]"=0.0, "2 Power [dBm]"=-33.0, "3 Freq. [MHz]"=0.0, "3 Power [dBm]"=-33.0}] ("Novatech settings") T4 [{"0 Freq. [MHz]"=139.72725, "0 Power [dBm]"=0.0, "Serial Port"="COM3", "1 Freq. [MHz]"=0.0, "1 Power [dBm]"=-33.0, "2 Freq. [MHz]"=35.0, "2 Power [dBm]"=-8.2, "3 Freq. [MHz]"=37.0, "3 Power [dBm]"=-6.7}, {"0 Freq. [MHz]"=0.0, "0 Power [dBm]"=-33.0, "Serial Port"="COM4", "1 Freq. [MHz]"=36.0, "1 Power [dBm]"=-8.2, "2 Freq. [MHz]"=40.0, "2 Power [dBm]"=-9.0, "3 Freq. [MHz]"=70.0, "3 Power [dBm]"=-0.5}, {"0 Freq. [MHz]"=86.0658125, "0 Power [dBm]"=0.0, "Serial Port"="COM5", "1 Freq. [MHz]"=0.0, "1 Power [dBm]"=-33.0, "2 Freq. [MHz]"=0.0, "2 Power [dBm]"=-33.0, "3 Freq. [MHz]"=0.0, "3 Power [dBm]"=-33.0}] ("Novatech settings")] -> w128
              frame "Manual" {
                n45 = local read "Novatech settings"() -> (w133:T4)
                n46 = local read "Master Output Bits"() -> (w130:bool[])
                n47 = local read "Slave Output Bits"() -> (w129:bool[])
                n48 = local read "DO Values"() -> (w132:T3)
                n49 = local read "AO Values"() -> (w131:T1)
              }
              frame "RbYb Warmup" {
                # "\"End on MOT\" but with shutters closed\n(Probe shutters OPEN)\n--CDH 1.3.12"
              }
              frame "RbYb Turn Off" {
                # "All currents off, shutters closed.\n--CDH 1.3.12"
              }
              frame "Yb MOT" {
                # "All currents off, shutters closed.\n--CDH 1.3.12"
              }
              frame "Rb MOT" {
              }
              frame "Sr Warmup" {
              }
            }
            n50 = local write "Master Output Bits"(w124) -> ()
            n51 = local write "Slave Output Bits"(w125) -> ()
            n52 = local write "Novatech settings"(w128) -> ()
            n53 = local write "AO Values"(w126) -> ()
            n54 = local write "DO Values"(w127) -> ()
          }
          event "Load": Value Change {
            n55 = event-data() -> ("NewVal"=w159:bool)  [unwired: 1 in, 4 out]
            n56 = case shown="True" w159 {
              frame False {
              }
              frame True {
                n57 = local read "Path"() -> (w164:path)
                n58 = local read "Master Output Bits"() -> (w187:bool[])
                n59 = local read "Novatech settings"() -> (w183:T4)
                n60 = property on="History" class="CmbBox"() -> ("Strings[]"=w190:string[])  [unwired: 2 in, 2 out]
                n61 = local read "Slave Output Bits"() -> (w186:bool[])
                n62 = local write "Load"(FALSE) -> ()
                n63 = local read "AO Values"() -> (w185:T1)
                n64 = local read "DO Values"() -> (w184:T3)
                n65 = Path To String(path=w164) -> (string=w189:string)
                n66 = Strip Path(path=w164) -> (name=w165:string)  [unwired: 1 out]
                n67 = call "Load_SetList_HistoryUpdate_v4.vi"("New Element"=w189, "History in"=w190) -> ()  [unwired: 1 out]
                n68 = call "Load_SetList_HistoryUpdate_v4.vi"("New Element"=w189, "History in"=w190) -> ("History Out"=w160:string[])
                n69 = property on="History" class="CmbBox"("Strings[]"=w160) -> ()  [unwired: 2 in, 2 out]
                n70 = Bundle("Master Output Bits"=w187, "Slave Output Bits"=w186, "AO Values"=w185, "DO Values"=w184, "Novatech settings"=w183) -> (w166:T9)  [unwired: 1 in]
                n71 = Concatenate Strings(w165, "_template") -> (w175:string)
                n72 = Build Path(base path=w164, name or relative path=w175) -> (appended path=w177:path)
                n73 = call <vilib>:"Open_Create_Replace File.vi"("file path"=w177) -> ("error out"=w167:errorcluster, "refnum"=w174:refnum<file>)  [unwired: 5 in, 4 out]
                n74 = Get File Size(file=w174, error in=w167) -> (refnum out=w173:refnum<file>, size (in bytes)=w171:i64, 0:w162:errorcluster)
                n75 = Unbundle By Name(w162) -> ("status"=w168:bool)
                n76 = To Long Integer(number=w171) -> (32bit integer=w172:i32)
                n77 = Equal To 0?(x=w172) -> (x = 0?=w169:bool)
                n78 = Or(x=w169, y=w168) -> (x .or. y?=w170:bool)
                n79 = case shown="False" w170 {
                  tunnel: [w194 w199] -> w163
                  tunnel: w166 -> [w195 w198]
                  tunnel: w173 -> [w196 w199]
                  tunnel: [w191 w198] -> w161
                  tunnel: w162 -> [w193 w197]
                  tunnel: [w192 w197] -> _
                  frame False {
                    # "Read out the data file"
                    n80 = Read from Binary File(5:w195, 8:w193, 11:w196) -> (0:w192:errorcluster, 2:w191:T9, 3:w194:refnum<file>)  [unwired: 4 out]
                  }
                  frame True {
                  }
                }
                n81 = Close File(refnum=w163) -> ()  [unwired: 1 in, 2 out]
                n82 = Unbundle(w161) -> ("Master Output Bits"=w182:bool[], "Slave Output Bits"=w181:bool[], "AO Values"=w180:T1, "DO Values"=w179:T3, "Novatech settings"=w178:T4)
                n83 = local write "Master Output Bits"(w182) -> ()
                n84 = local write "Slave Output Bits"(w181) -> ()
                n85 = local write "Novatech settings"(w178) -> ()
                n86 = local write "AO Values"(w180) -> ()
                n87 = local write "DO Values"(w179) -> ()
              }
            }
          }
          event "Save": Value Change {
            n88 = event-data() -> ("NewVal"=w200:bool)  [unwired: 1 in, 4 out]
            n89 = case shown="True" w200 {
              frame False {
              }
              frame True {
                n90 = local read "Path"() -> (w204:path)
                n91 = property on="History" class="CmbBox"() -> ("Strings[]"=w220:string[])  [unwired: 2 in, 2 out]
                n92 = local write "Save"(FALSE) -> ()
                n93 = Path To String(path=w204) -> (string=w219:string)
                n94 = call "Load_SetList_HistoryUpdate_v4.vi"("New Element"=w219, "History in"=w220) -> ()  [unwired: 1 out]
                n95 = call "Load_SetList_HistoryUpdate_v4.vi"("New Element"=w219, "History in"=w220) -> ("History Out"=w201:string[])
                n96 = property on="History" class="CmbBox"("Strings[]"=w201) -> ()  [unwired: 2 in, 2 out]
                n97 = Create Folder(path (use dialog)=w204) -> (created path=w203:path)  [unwired: 1 in, 3 out]
                n98 = Strip Path(path=w204) -> (name=w205:string)  [unwired: 1 out]
                n99 = local read "Master Output Bits"() -> (w217:bool[])
                n100 = local read "Novatech settings"() -> (w213:T4)
                n101 = local read "Slave Output Bits"() -> (w216:bool[])
                n102 = local read "AO Values"() -> (w215:T1)
                n103 = local read "DO Values"() -> (w214:T3)
                n104 = Concatenate Strings(w205, "_template") -> (w207:string)
                n105 = Build Path(base path=w203, name or relative path=w207) -> (appended path=w211:path)
                n106 = call <vilib>:"Open_Create_Replace File.vi"("function (open:0)"=T6."create or replace", "file path"=w211) -> ("refnum"=w212:refnum<file>)  [unwired: 4 in, 5 out]
                n107 = Bundle("Master Output Bits"=w217, "Slave Output Bits"=w216, "AO Values"=w215, "DO Values"=w214, "Novatech settings"=w213) -> (w202:T9)  [unwired: 1 in]
                n108 = Write to Binary File(file (use dialog)=w212, data=w202, 5:TRUE ("prepend array or string size? (T)")) -> (refnum out=w209:refnum<file>)  [unwired: 1 in, 4 out]
                n109 = Close File(refnum=w209) -> ()  [unwired: 1 in, 2 out]
              }
            }
          }
        }
      }
    }
  }
  n110 = call <vilib>:"Release Semaphore_71.vi"("error in (no error)"=w9, "semaphore"=w1) -> ("error out"=w10:errorcluster, "semaphore out"=w11:T5)  [unwired: 4 out]
  n111 = call <vilib>:"Destroy Semaphore.vi"("error in (no error)"=w10, "semaphore"=w11) -> ("error out"=→"error out":errorcluster)  [unwired: 5 out]
